vi "Read Poll Interval (ms).vi"(8 "error in (no error)":errorcluster, 11 "Polled_EventSource in":refnum<class "Polled_EventSource.lvclass">) -> (0 "error out":errorcluster, 2 "Poll Interval (ms)":i32=10, 3 "Polled_EventSource out":refnum<class "Polled_EventSource.lvclass">)   [LabVIEW 2021, in "Polled_EventSource.lvclass"]
uses:
  Polled_EventSource.lvclass
  Polled_EventSource.lvclass/Polled_EventSource.ctl
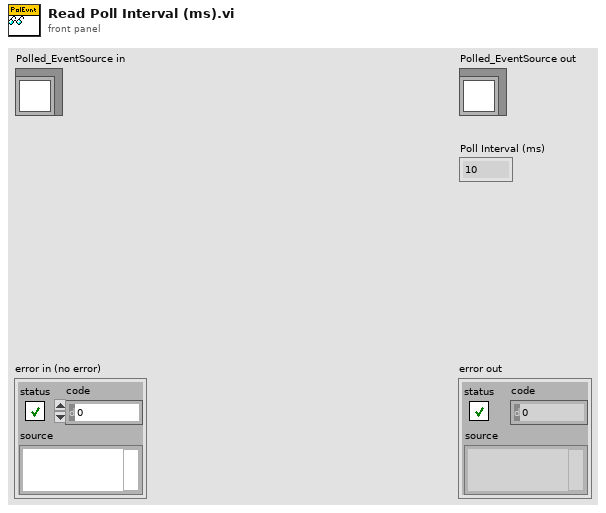
[diagram p1: front panel]
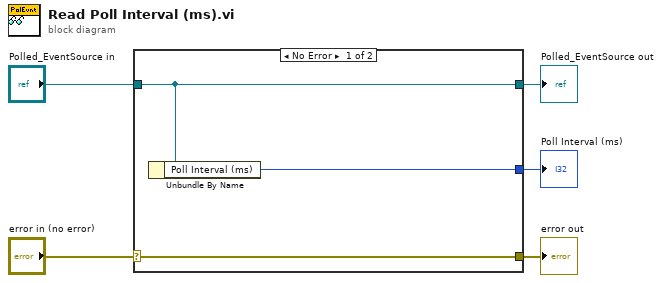
[diagram p0: block diagram]
diagram:
  n1 = case shown="No Error" "error in (no error)" {
    selector: "error in (no error)" -> [w8 w9]
    tunnel: [w8 w9] -> w4
    tunnel: [w7 w10] -> w2
    tunnel: "Polled_EventSource in" -> [w7 w10]
    tunnel: [w6 _] -> w1
    frame No Error {
      n2 = Unbundle By Name(w7) -> ("Poll Interval (ms)"=w6:i32)
    }
    frame Error {
    }
  }
  "error out" <- w4
  "Polled_EventSource out" <- w2
  "Poll Interval (ms)" <- w1
